vi "Find Component in Component List.vi"(3 "Component Id":u8=1, 5 "ComponentSeq":T1[](array[typedef])) -> (0 "Record Exists?":bool, 1 "ComponentRec":T1={"Component Id"=1, "Instance Id"=0, "ServiceSeq"=[{"ServiceURI"="1", "MajorVerNum"=1, "MinorVerNum"=1}]}, 2 "Component Index":i32)   [LabVIEW 2009]
uses:
  ComponentRec.ctl
  ServiceRec.ctl
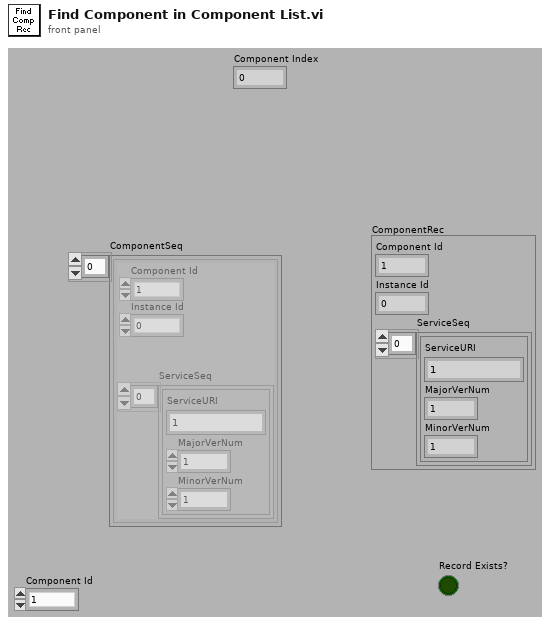
[diagram p1: front panel]
types:
  T1 = typedef "ComponentRec.ctl" = cluster{"Component Id":u8, "Instance Id":u8, "ServiceSeq":T2[]}
  T2 = typedef "ServiceRec.ctl" = cluster{"ServiceURI":string, "MajorVerNum":u8, "MinorVerNum":u8}
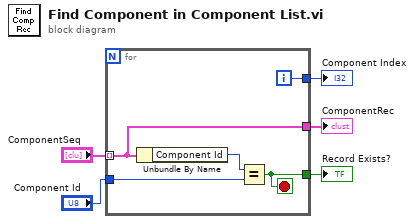
[diagram p0: block diagram]
diagram:
  n1 = for {
    tunnel: "ComponentSeq" -> [w8] mode=indexing
    tunnel: "Component Id" -> [w9]
    tunnel: [w8] -> w3
    tunnel: [w7] -> w2
    tunnel: [w6] -> w1
    i -> [w6]
    stop <- w7 stop-if-true
    n2 = Unbundle By Name(w8) -> ("Component Id"=w10:u8)
    n3 = Equal?(x=w10, y=w9) -> (x = y?=w7:bool)
  }
  "ComponentRec" <- w3
  "Record Exists?" <- w2
  "Component Index" <- w1
